vi "Save data file to network drive v1.vi"(11 "panel id":string) -> (0 "network file save error":errorcluster)   [LabVIEW 2013]
uses:
  Global 1.vi
panel:
  out "network file dir path":path
  out "network dir":string
  out "file save path":string
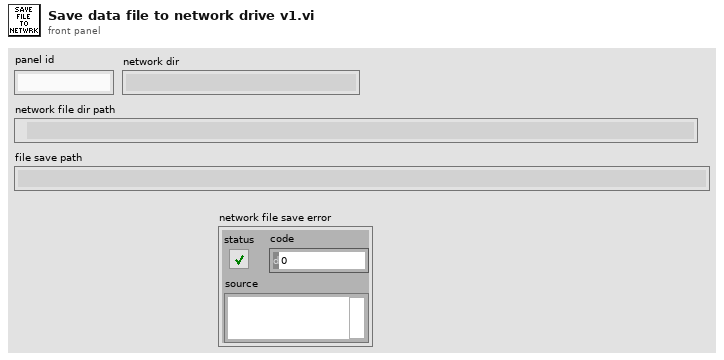
[diagram p1: front panel]
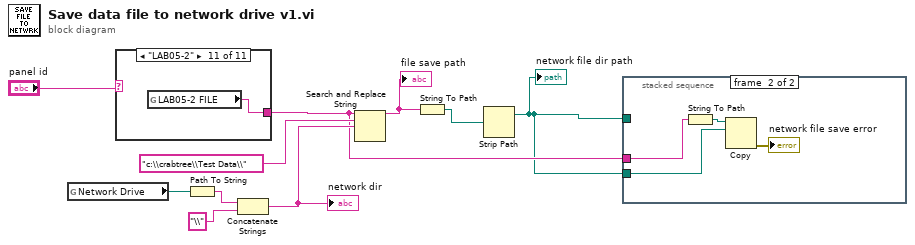
[diagram p0: block diagram]
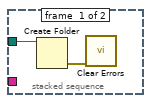
[diagram p2: hidden frame]
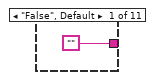
[diagram p3: hidden frame]
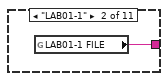
[diagram p4: hidden frame]
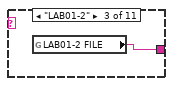
[diagram p5: hidden frame]
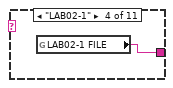
[diagram p6: hidden frame]
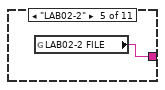
[diagram p7: hidden frame]
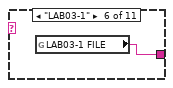
[diagram p8: hidden frame]
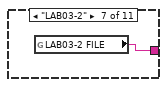
[diagram p9: hidden frame]
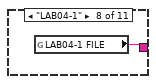
[diagram p10: hidden frame]
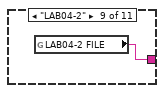
[diagram p11: hidden frame]
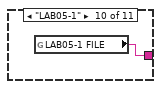
[diagram p12: hidden frame]
diagram:
  n1 = global read "Global 1.vi" "Network Drive"() -> (w8:path)
  n2 = case shown="\"LAB05-2\"" "panel id" {
    tunnel: ["" w12 w13 w14 w15 w16 w17 w18 w19 w20 w21] -> w2
    frame "False", Default {
    }
    frame "LAB01-1" {
      n3 = global read "Global 1.vi" "LAB01-1 FILE"() -> (w12:string)
    }
    frame "LAB01-2" {
      n4 = global read "Global 1.vi" "LAB01-2 FILE"() -> (w13:string)
    }
    frame "LAB02-1" {
      n5 = global read "Global 1.vi" "LAB02-1 FILE"() -> (w14:string)
    }
    frame "LAB02-2" {
      n6 = global read "Global 1.vi" "LAB02-2 FILE"() -> (w15:string)
    }
    frame "LAB03-1" {
      n7 = global read "Global 1.vi" "LAB03-1 FILE"() -> (w16:string)
    }
    frame "LAB03-2" {
      n8 = global read "Global 1.vi" "LAB03-2 FILE"() -> (w17:string)
    }
    frame "LAB04-1" {
      n9 = global read "Global 1.vi" "LAB04-1 FILE"() -> (w18:string)
    }
    frame "LAB04-2" {
      n10 = global read "Global 1.vi" "LAB04-2 FILE"() -> (w19:string)
    }
    frame "LAB05-1" {
      n11 = global read "Global 1.vi" "LAB05-1 FILE"() -> (w20:string)
    }
    frame "LAB05-2" {
      n12 = global read "Global 1.vi" "LAB05-2 FILE"() -> (w21:string)
    }
  }
  n13 = Path To String(path=w8) -> (string=w7:string)
  n14 = Concatenate Strings(w7, "\\") -> (w5:string)
  "network dir" <- w5
  n15 = Search and Replace String(input string=w2, search string="c:\\crabtree\\Test Data\\", replace string=w5) -> (result string=w4:string)  [unwired: 5 in, 3 out]
  "file save path" <- w4
  n16 = String To Path(string=w4) -> (path=w3:path)
  n17 = Strip Path(path=w3) -> (stripped path=w1:path)  [unwired: 1 out]
  "network file dir path" <- w1
  n18 = stacked-sequence {
    tunnel: w1 -> [w23 _]
    tunnel: w2 -> [_ w25]
    tunnel: w1 -> [_ w24]
    frame #0 {
      n19 = Create Folder(path (use dialog)=w23) -> (error out=w22:errorcluster)  [unwired: 2 in, 2 out]
      n20 = call <vilib>:"Clear Errors.vi"("error in (no error)"=w22) -> ()  [unwired: 6 in, 1 out]
    }
    frame #1 {
      n21 = String To Path(string=w25) -> (path=w26:path)
      n22 = Copy(10:w24, 11:w26) -> (0:→"network file save error":errorcluster)  [unwired: 3 in, 2 out]
    }
  }
